vi "Post-Project-Copying Process.vi"(10 "MetaDataObj":refnum<class "MetaDataObj.lvclass">) -> ()   [LabVIEW 2021, in "Plugin Generator.lvlib"]
uses:
  Plugin Generator.lvlib
  ed511516-c131-45ea-930f-d7c7c2eb0895.vi
  <resource>/dialog/NewProjectWizard/MetaDataObj/MetaDataObj.lvclass
panel:
  out "To display":string="All Process Done. The Project Root will pop up later."
  out "Progress":string
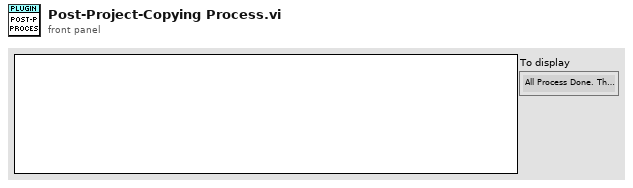
[diagram p1: front panel]
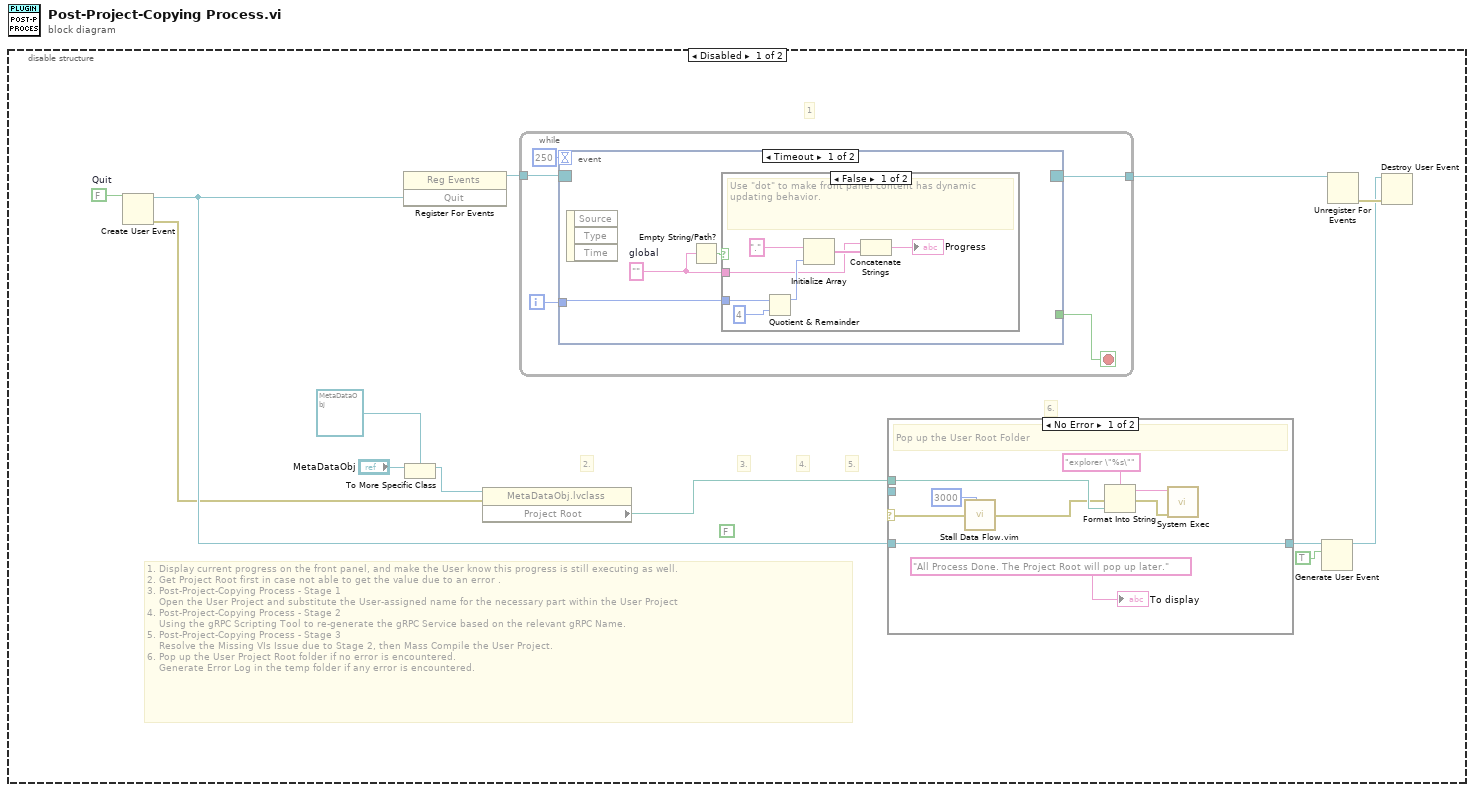
[diagram p0: block diagram]
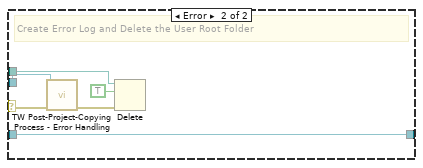
[diagram p2: hidden frame]
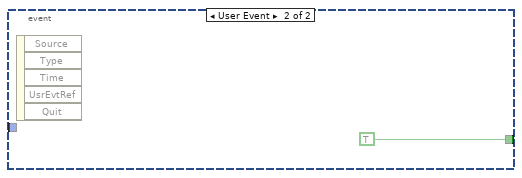
[diagram p4: hidden frame]
diagram:
  n1 = disable-structure shown="Disabled" {
    frame Disabled {
      w12 = FALSE  # Quit
      (unwired) FALSE ("Debug")
      # "6."
      # "5."
      # "4."
      # "3."
      # "1. Display current progress on the front panel, and make the User know this progress is still executing as well.\n2. Get Project Root first in case not able to get the value due to an error .\n3. Post-Project-Copying Process - Stage 1\n    Open the User Project and substitute the User-assigned name for the necessary part within the User Project\n4. Post-Project-Copying Process - Stage 2\n    Using the gRPC Scripting Tool to re-generate the gRPC Service based on the relevant gRPC Name.\n5. Post-Project-Copying Process - Stage 3\n    Resolve the Missing VIs Issue due to Stage 2, then Mass Compile the User Project.\n6. Pop up the User Project Root folder if no error is encountered.\n    Generate Error Log in the temp folder if any error is encountered."
      # "2."
      # "1"
      n2 = Create User Event(user event datatype=w12) -> (user event=w5:refnum<user-event>, error out=w3:errorcluster)  [unwired: 1 in]
      n3 = register-events(w5) -> (reference out=w11:refnum<event-registration>)  [unwired: 2 in, 1 out]
      n4 = To More Specific Class(target class=refnum<class "MetaDataObj.lvclass"> refnum ("MetaDataObj"), reference="MetaDataObj") -> (specific class reference=w4:refnum<class "MetaDataObj.lvclass">)  [unwired: 1 in, 1 out]
      n5 = property class="MetaDataObj.lvclass"(reference=w4, error in=w3) -> ("Project Root"=w2:path)  [unwired: 2 out]
      n6 = while {
        tunnel: w11 -> [w32]
        tunnel: [w29] -> w9
        i -> [w30]
        stop <- w31 stop-if-true
        n7 = event shown="[0] Timeout" {
          selector: w32 -> [_ _]
          dyn-events: [_ _] -> w29
          timeout: 250 -> [_ _]
          tunnel: [_ TRUE] -> w31
          tunnel: w30 -> [w35 _]
          event Timeout {
            w34 = ""  # global
            n8 = event-data() -> ()  [unwired: 1 in, 3 out]
            n9 = Empty String/Path?(string/path=w34) -> (empty?=w36:bool)
            n10 = case shown="False" w36 {
              tunnel: w34 -> [w40 _]
              tunnel: w35 -> [w38 _]
              frame False {
                # "Use \"dot\" to make front panel content has dynamic updating behavior."
                n11 = Quotient & Remainder(x=w38, y=4) -> (x-y*floor(x/y)=w43:i32)  [unwired: 1 out]
                n12 = Initialize Array(".", w43) -> (w41:string[])
                n13 = Concatenate Strings(w40, w41) -> (→"Progress":string)
              }
              frame True {
                # "No dynamic update front panel content due to progress not starting yet."
              }
            }
          }
          event User Event {
            n14 = event-data() -> ()  [unwired: 1 in, 5 out]
          }
        }
      }
      n15 = case shown="No Error" {
        selector: _ -> [w17 w27]
        tunnel: [w19 w28] -> w6
        tunnel: w5 -> [w19 w28]
        tunnel: w2 -> [w18 w24]
        tunnel: _ -> [_ w26]
        frame No Error {
          # "Pop up the User Root Folder"
          n16 = call "Stall Data Flow.vim"("value in"=w17, "milliseconds to wait"=u32 3000) -> ("value out"=w16:errorcluster)  [unwired: 1 out]
          n17 = Format Into String(format string="explorer \"%s\"", error in=w16, w18) -> (resulting string=w22:string, error out=w20:errorcluster)  [unwired: 1 in]
          n18 = call <vilib>:"System Exec.vi"("error in (no error)"=w20, "command line"=w22) -> ()  [unwired: 6 in, 4 out]
          "To display" <- "All Process Done. The Project Root will pop up later." ("Progress")
        }
        frame Error {
          # "Create Error Log and Delete the User Root Folder"
          n19 = call "TW Post-Project-Copying Process - Error Handling.vi"("error in"=w27, 11:w26) -> ("error out"=w25:errorcluster)  [unwired: 9 in]
          n20 = Delete(path (use dialog)=w24, entire hierarchy (F)=TRUE, error in=w25) -> ()  [unwired: 2 in, 3 out]
        }
      }
      n21 = Generate User Event(user event=w6, event data cluster=TRUE ("event data")) -> (user event out=w7:refnum<user-event>)  [unwired: 2 in, 1 out]
      n22 = Unregister For Events(event registration refnum=w9) -> (error out=w8:errorcluster)  [unwired: 1 in]
      n23 = Destroy User Event(user event=w7, error in=w8) -> ()  [unwired: 1 out]
    }
    frame Enabled {
    }
  }
